vi "DisplayPanel.vi"() -> ()   [LabVIEW 2013]
uses:
  MvLVLib/MvCameraControl.lvlib
  MvLVLib/VIs/CreateGigEHandle.vi
  MvLVLib/VIs/CreateU3VHandle.vi
panel:
  out "GenTLDeviceArray":T1(array[cluster])
  out "Image":T2(plugin-control)
  out "U3VDeviceArray":T3(array[cluster])
  out "GigEDeviceArray":T4(array[cluster])
  in  "pConvertInfo In":T5
  out "PixelFormat":u32
  out "handle out":u64
  out "PayloadSize":u32
  out "pFrameInfoEx out":T6
  out "nHeight":u32
  out "nWidth":u32
  out "Acquisision Flag":bool
  in  "Trigger Mode":bool
  in  "Continuous":bool
  out "打开标志":bool
  in  "stop":bool
  in  "Trigger Once":bool
  in  "Stop":bool
  in  "Start":bool
  in  "Open Device":bool
  in  "Close Device":bool
  in  "error in (no error) 2":errorcluster caption="错误输入（无错误）"
  in  "Refresh Devices":bool
  in  "Device List":u16(ring)
  # "Initialize"
  # "Acquisition"
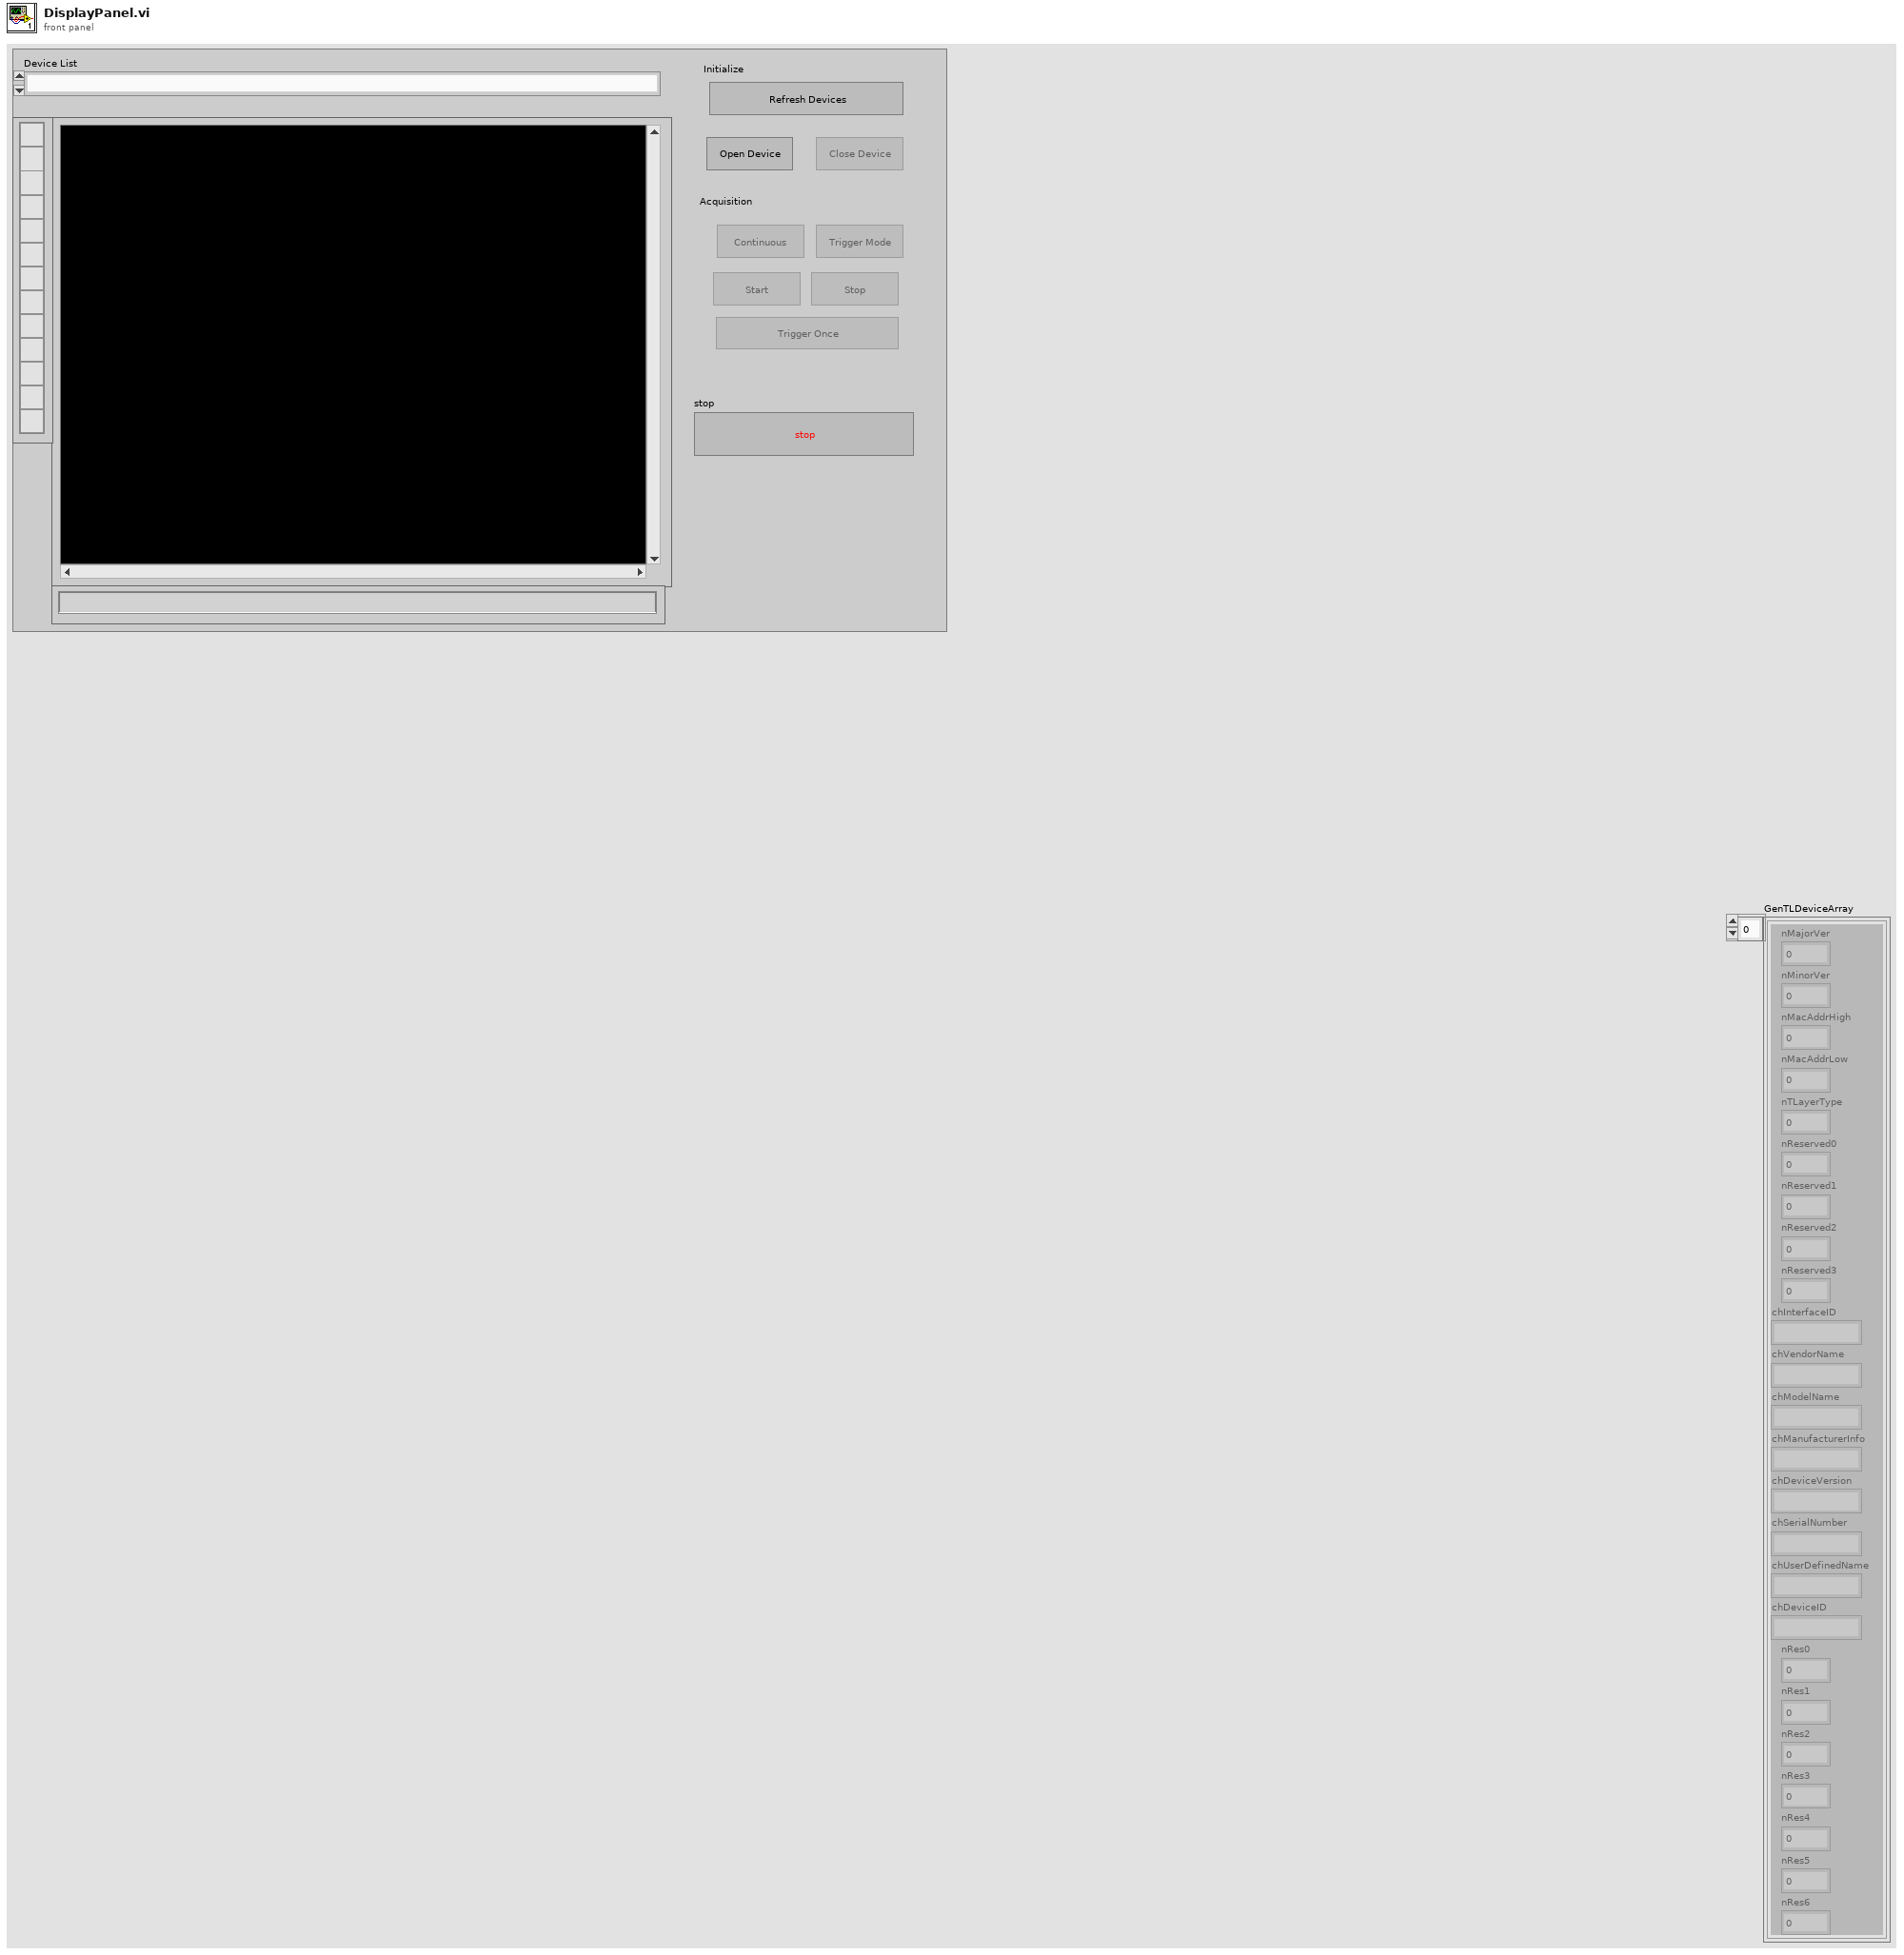
[diagram p1: front panel]
types:
  T1 = cluster{"nMajorVer":u16, "nMinorVer":u16, "nMacAddrHigh":u32, "nMacAddrLow":u32, "nTLayerType":u32, "nReserved0":u32, "nReserved1":u32, "nReserved2":u32, "nReserved3":u32, "chInterfaceID":string, "chVendorName":string, "chModelName":string, "chManufacturerInfo":string, "chDeviceVersion":string, "chSerialNumber":string, "chUserDefinedName":string, "chDeviceID":string, "nRes0":u32, "nRes1":u32, "nRes2":u32, "nRes3":u32, "nRes4":u32, "nRes5":u32, "nRes6":u32}[]
  T2 = typedef "IMAQ Image.ctl" = refnum<image>
  T3 = cluster{"nMajorVer":u16, "nMinorVer":u16, "nMacAddrHigh":u32, "nMacAddrLow":u32, "nTLayerType":u32, "nReserved0":u32, "nReserved1":u32, "nReserved2":u32, "nReserved3":u32, "CrtlInEndPoint":u8, "CrtlOutEndPoint":u8, "StreamEndPoint":u8, "EventEndPoint":u8, "idVendor":u16, "idProduct":u16, "nDeviceNumber":u32, "chDeviceGUID":string, "chVendorName":string, "chModelName":string, "chFamilyName":string, "chDeviceVersion":string, "chManufacturerName":string, "chSerialNumber":string, "chUserDefinedName":string, "nbcdUSB":u32, "nDeviceAddress":u32, "nRes0":u32, "nRes1":u32, "nResAlign":u32}[]
  T4 = cluster{"nMajorVer":u16, "nMinorVer":u16, "nMacAddrHigh":u32, "nMacAddrLow":u32, "nTLayerType":u32, "nReserved0":u32, "nReserved1":u32, "nReserved2":u32, "nReserved3":u32, "nIpCfgOption":u32, "nIpCfgCurrent":u32, "nCurrentIp":u32, "nCurrentSubNetMask":u32, "nDefaultGateWay":u32, "chManualfacturerName":string, "chModelName":string, "chDeviceVersion":string, "chManufacturerSpecificInfo":string, "chSerialNumber":string, "chUserDefinedName":string, "nNetExport":u32, "nRes0":u32, "nRes1":u32, "nRes2":u32, "nRes3":u32}[]
  T5 = cluster{"nWidth":u16, "nHeight":u16, "enSrcPixelType":u32, "nSrcDataLen":u32, "enDstPixelType":u32, "nDstLen":u32, "nDstBufferSize":u32, "nRes0":u32, "nRes1":u32, "nRes2":u32, "nRes3":u32}
  T6 = cluster{"nWidth":u16, "nHeight":u16, "enPixelType":i32, "nFrameNum":u32, "nDevTimeStampHigh":u32, "nDevTimeStampLow":u32, "nReserved0":u32, "nHostTimeStamp":i64, "nFrameLen":u32, "nSecondCount]":u32, "nCycleCount":u32, "nCycleOffset":u32, "fGain":u32, "fExposureTime":u32, "nAverageBrightness":u32, "nRed":u32, "nGreen":u32, "nBlue":u32, "nFrameCounter":u32, "nTriggerIndex":u32, "nInput":u32, "nOutput":u32, "nOffsetX":u32, "nOffsetY":u32, "nReserved[0]":u32, "nReserved[1]":u32, "nReserved[2]":u32, "nReserved[3]":u32, "nReserved[4]":u32, "nReserved[5]":u32, "nReserved[6]":u32, "nReserved[7]":u32, "nReserved[8]":u32, "nReserved[9]":u32, "nReserved[10]":u32, "nReserved[11]":u32, "nReserved[12]":u32, "nReserved[13]":u32, "nReserved[14] 10":u32, "nReserved[15] 11":u32, "nReserved[16] 12":u32, "nReserved[17] 13":u32, "nReserved[18] 14":u32, "nReserved[19] 15":u32, "nReserved[20] 16":u32, "nReserved[21] 17":u32, "nReserved[22] 18":u32, "nReserved[23] 19":u32, "nReserved[24] 20":u32, "nReserved[25] 21":u32, "nReserved[26] 22":u32, "nReserved[27] 23":u32, "nReserved[28] 24":u32, "nReserved[29] 25":u32, "nReserved[30] 26":u32, "nReserved[31] 27":u32, "nReserved[32] 28":u32, "nReserved[33] 29":u32, "nReserved[34] 30":u32, "nReserved[35] 31":u32, "nReserved[36] 32":u32, "nReserved[37] 33":u32, "nReserved[38] 34":u32, "nReserved[39] 35":u32, "nReserved[40] 36":u32}
  T7 = enum8{"Enabled", "Disabled", "Disabled and Grayed Out"}
  T8 = cluster{"nMajorVer":u16, "nMinorVer":u16, "nMacAddrHigh":u32, "nMacAddrLow":u32, "nTLayerType":u32, "nReserved0":u32, "nReserved1":u32, "nReserved2":u32, "nReserved3":u32, "nIpCfgOption":u32, "nIpCfgCurrent":u32, "nCurrentIp":u32, "nCurrentSubNetMask":u32, "nDefaultGateWay":u32, "chManualfacturerName":string, "chModelName":string, "chDeviceVersion":string, "chManufacturerSpecificInfo":string, "chSerialNumber":string, "chUserDefinedName":string, "nNetExport":u32, "nRes0":u32, "nRes1":u32, "nRes2":u32, "nRes3":u32}
  T9 = cluster{"nMajorVer":u16, "nMinorVer":u16, "nMacAddrHigh":u32, "nMacAddrLow":u32, "nTLayerType":u32, "nReserved0":u32, "nReserved1":u32, "nReserved2":u32, "nReserved3":u32, "CrtlInEndPoint":u8, "CrtlOutEndPoint":u8, "StreamEndPoint":u8, "EventEndPoint":u8, "idVendor":u16, "idProduct":u16, "nDeviceNumber":u32, "chDeviceGUID":string, "chVendorName":string, "chModelName":string, "chFamilyName":string, "chDeviceVersion":string, "chManufacturerName":string, "chSerialNumber":string, "chUserDefinedName":string, "nbcdUSB":u32, "nDeviceAddress":u32, "nRes0":u32, "nRes1":u32, "nResAlign":u32}
  T10 = cluster{"nCurValue":u32, "nMax":u32, "nMin":u32, "nInc":u32, "nReserved[0]":u32, "nReserved[1]":u32, "nReserved[2]":u32, "nReserved[3]":u32}
  T11 = cluster{"nCurValue":u32, "nSupportedNum":u32, "nSupportValue":u32[], "nReserved[0]":u32, "nReserved[1]":u32, "nReserved[2]":u32, "nReserved[3]":u32}
  T12 = cluster{"nWidth":u32, "nHeight":u32, "enSrcPixelType":u32, "nSrcDataLen":u32, "enDstPixelType":u32, "nDstLen":u32, "nDstBufferSize":u32, "nRes0":u32, "nRes1":u32, "nRes2":u32, "nRes3":u32}
  T13 = typedef "Image Type" = u32
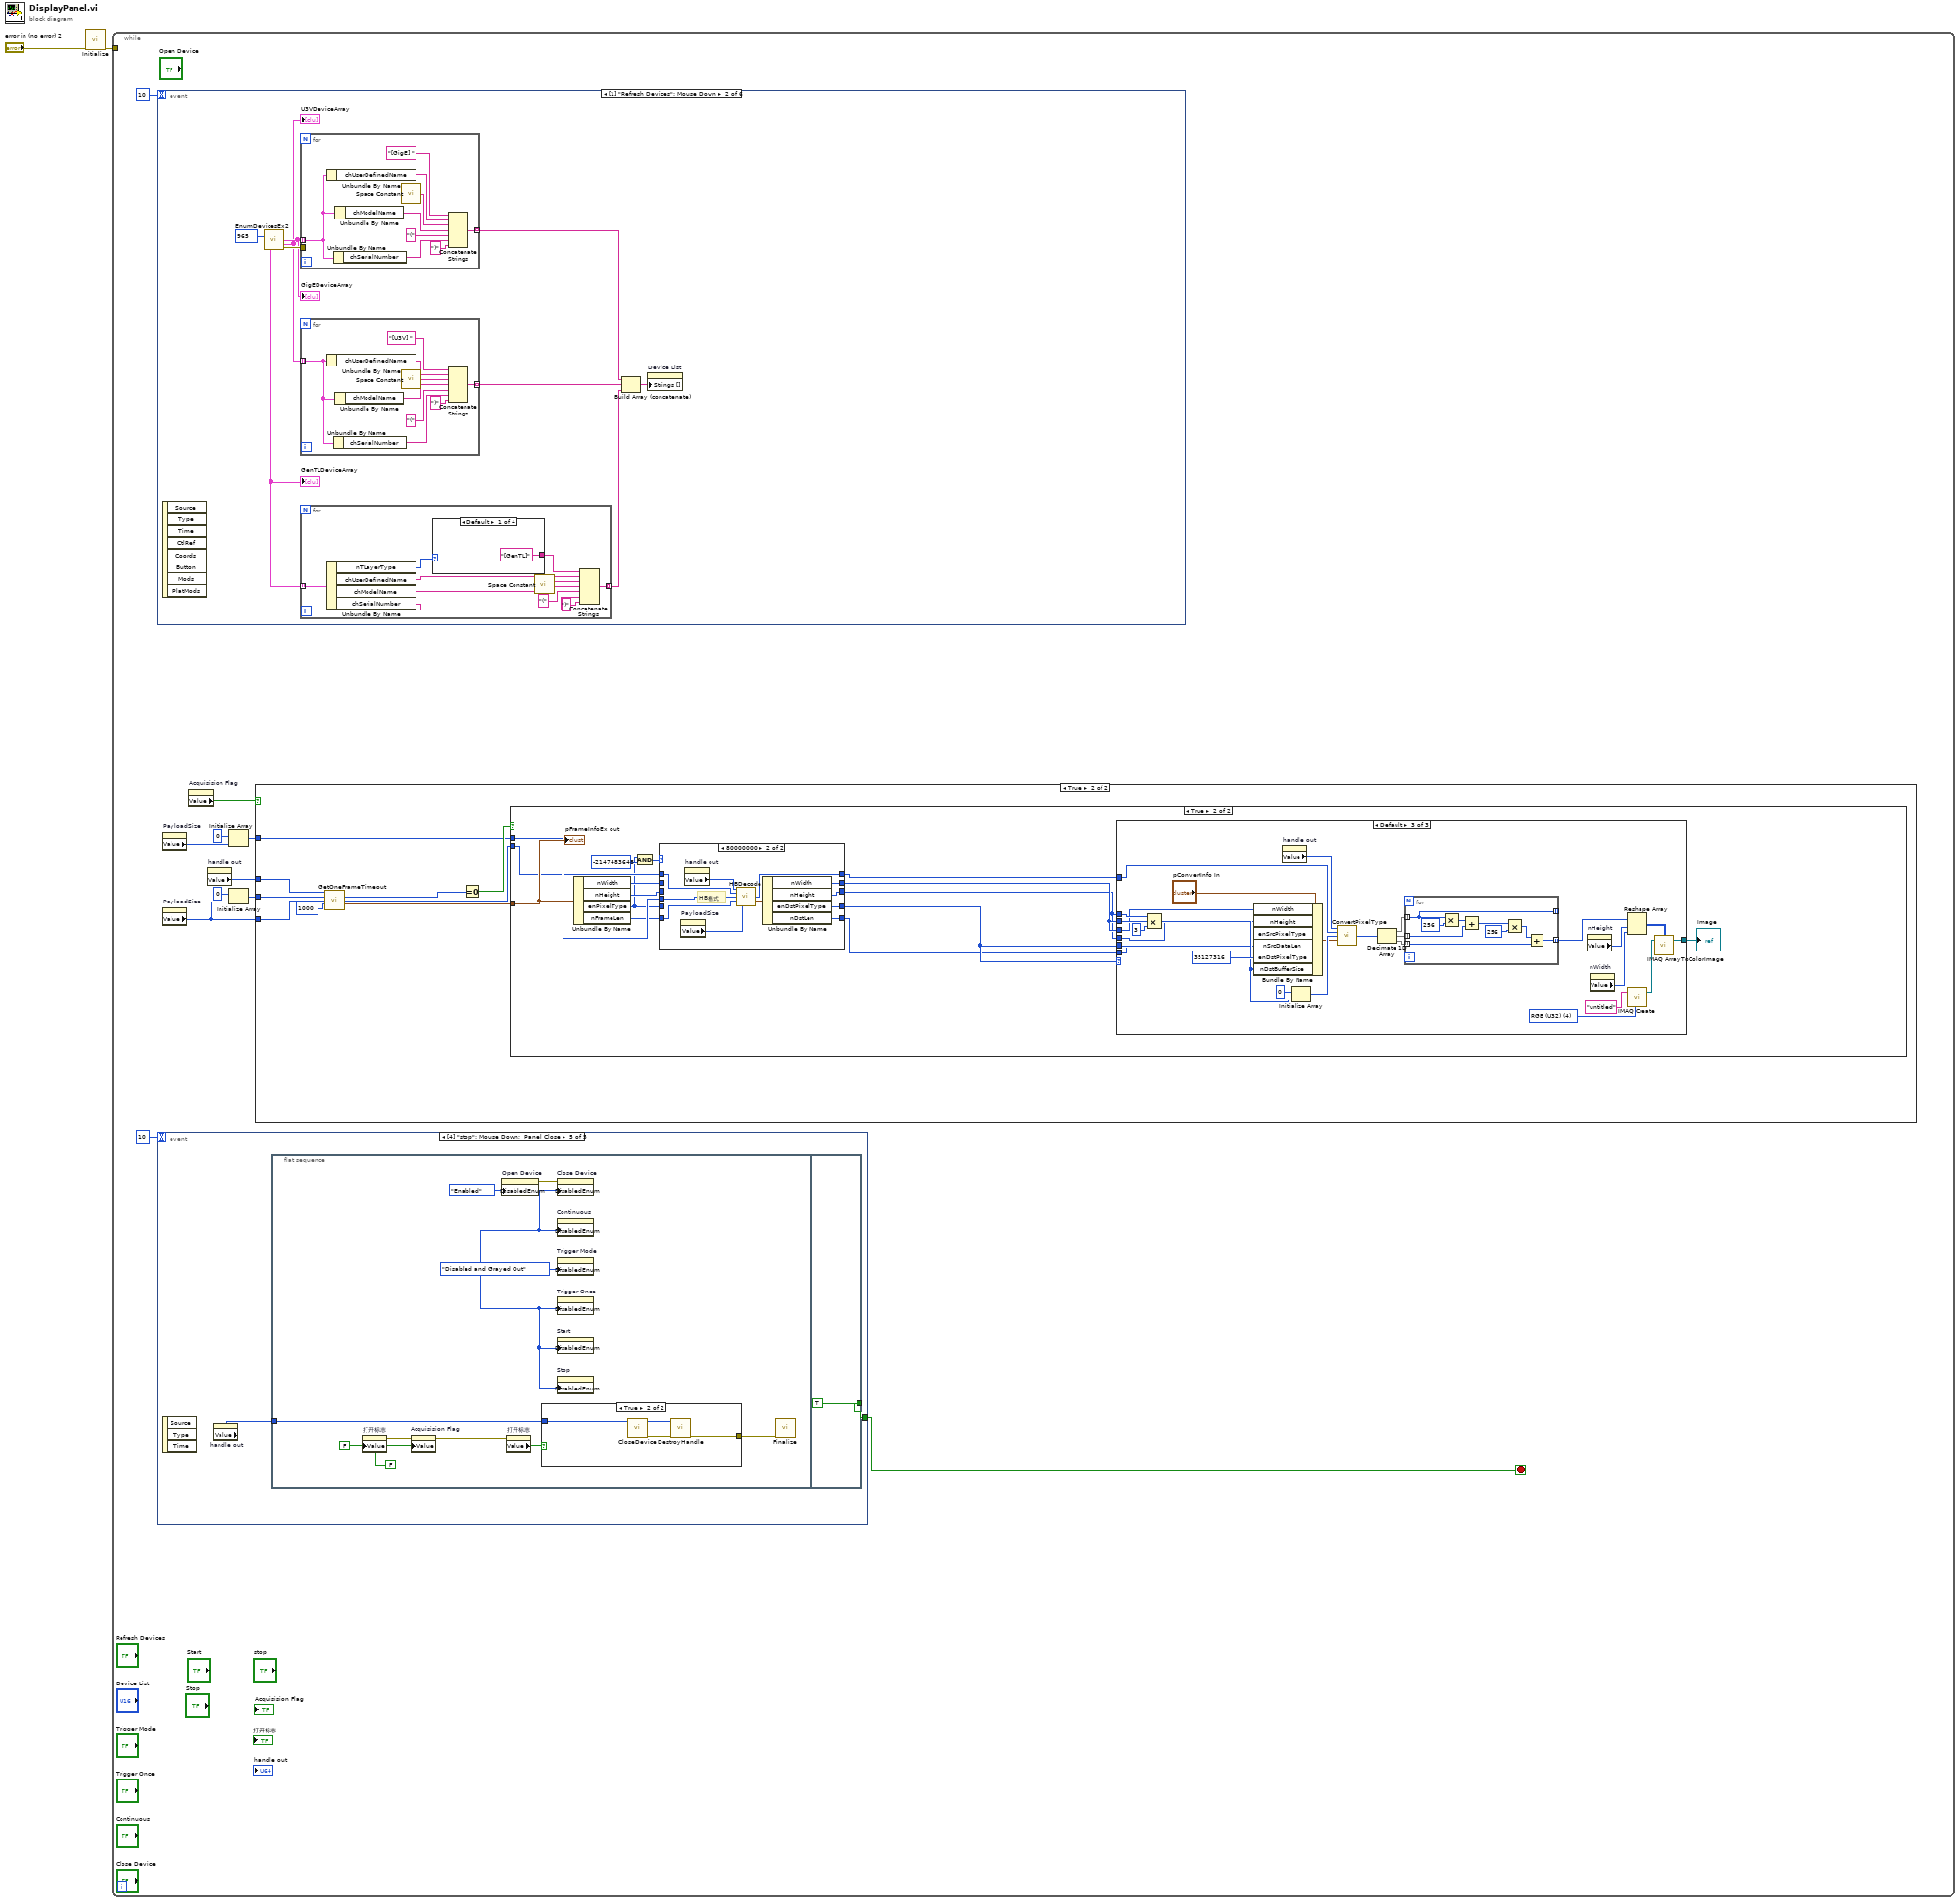
[diagram p0: block diagram]
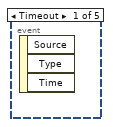
[diagram p2: hidden frame]
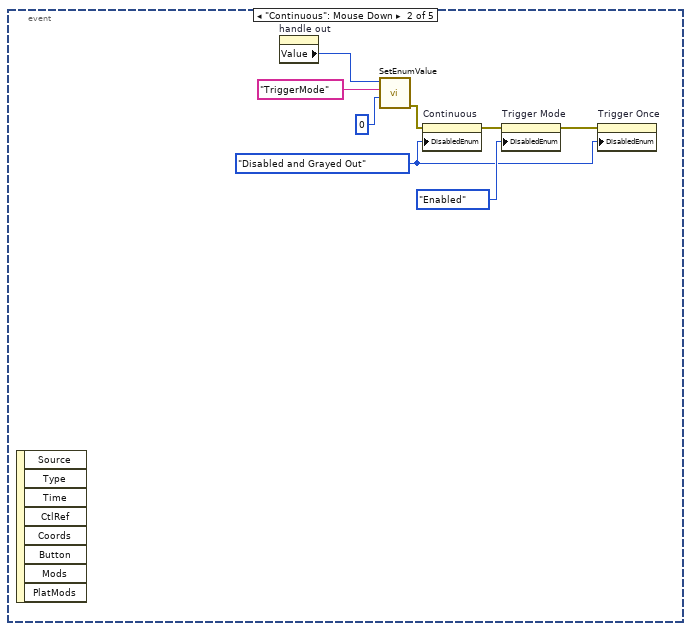
[diagram p3: hidden frame]
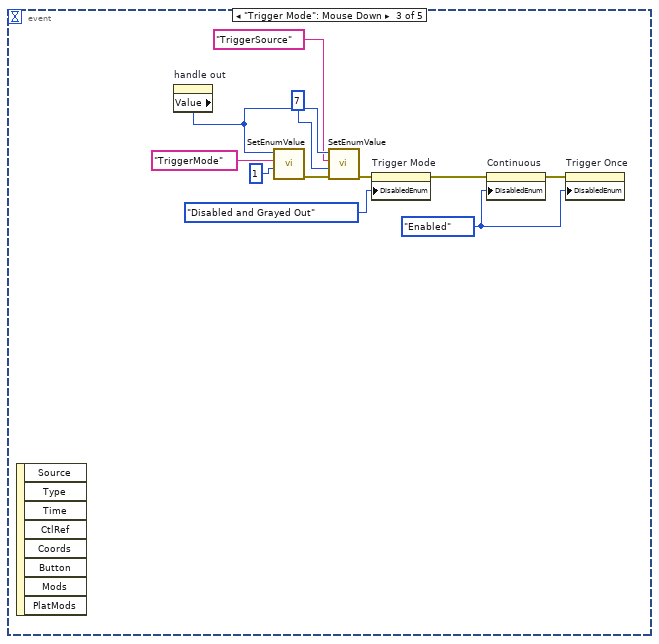
[diagram p4: hidden frame]
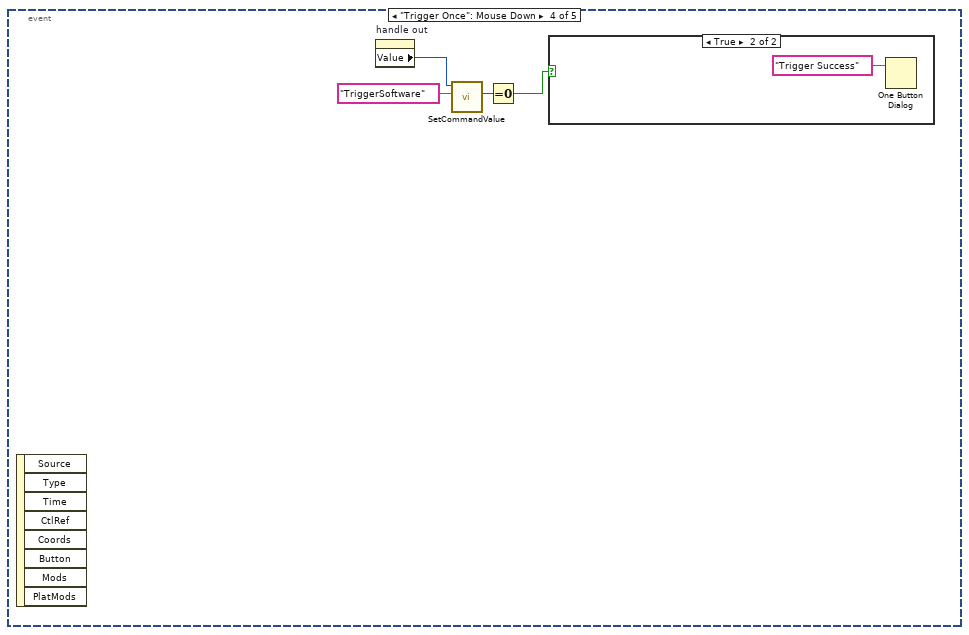
[diagram p5: hidden frame]
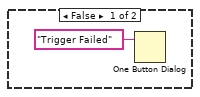
[diagram p6: hidden frame]
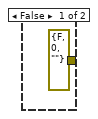
[diagram p7: hidden frame]
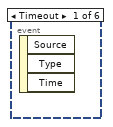
[diagram p8: hidden frame]
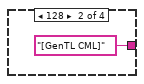
[diagram p9: hidden frame]
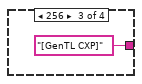
[diagram p10: hidden frame]
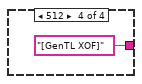
[diagram p11: hidden frame]
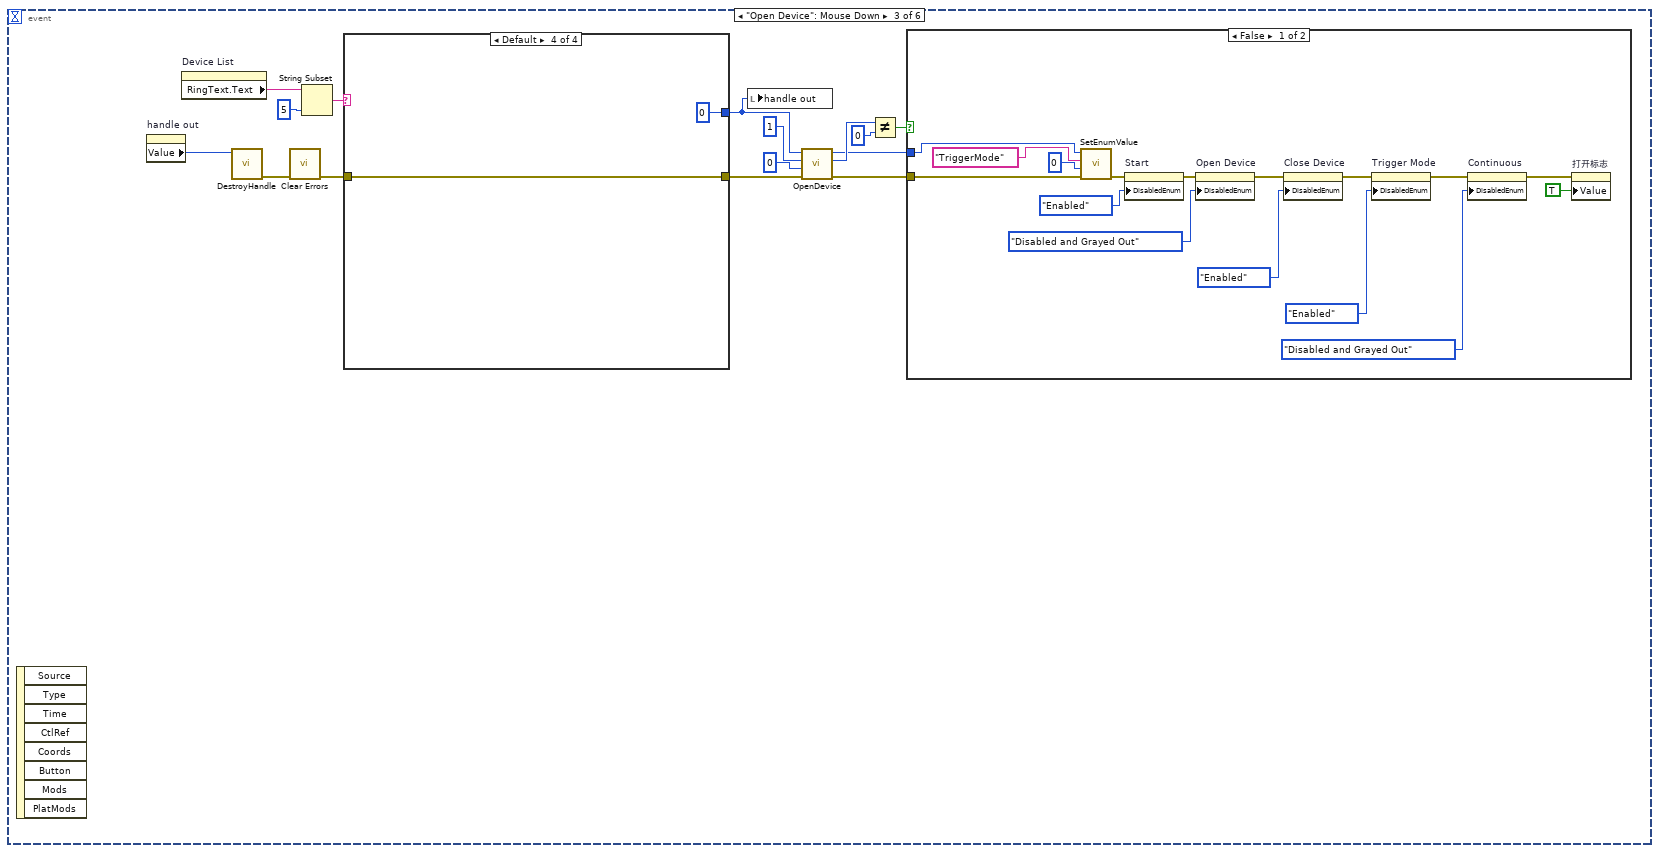
[diagram p12: hidden frame]
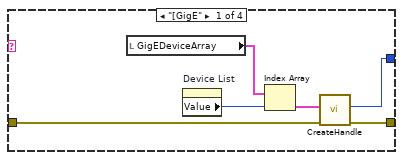
[diagram p13: hidden frame]
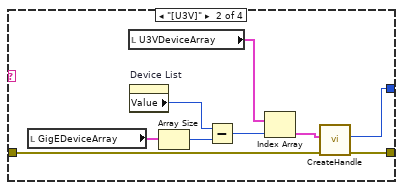
[diagram p14: hidden frame]
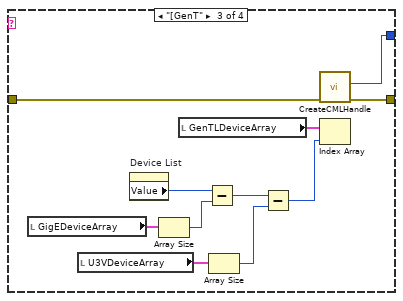
[diagram p15: hidden frame]
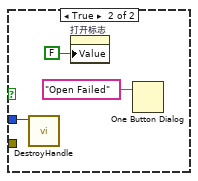
[diagram p16: hidden frame]
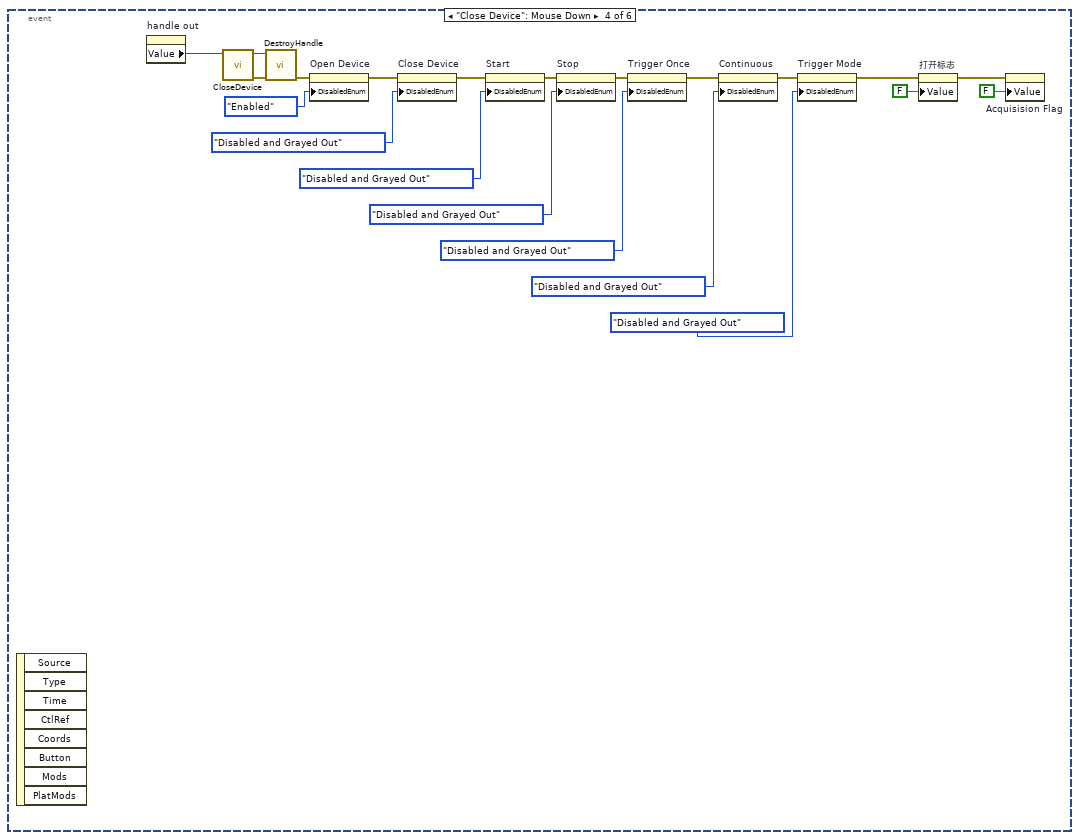
[diagram p17: hidden frame]
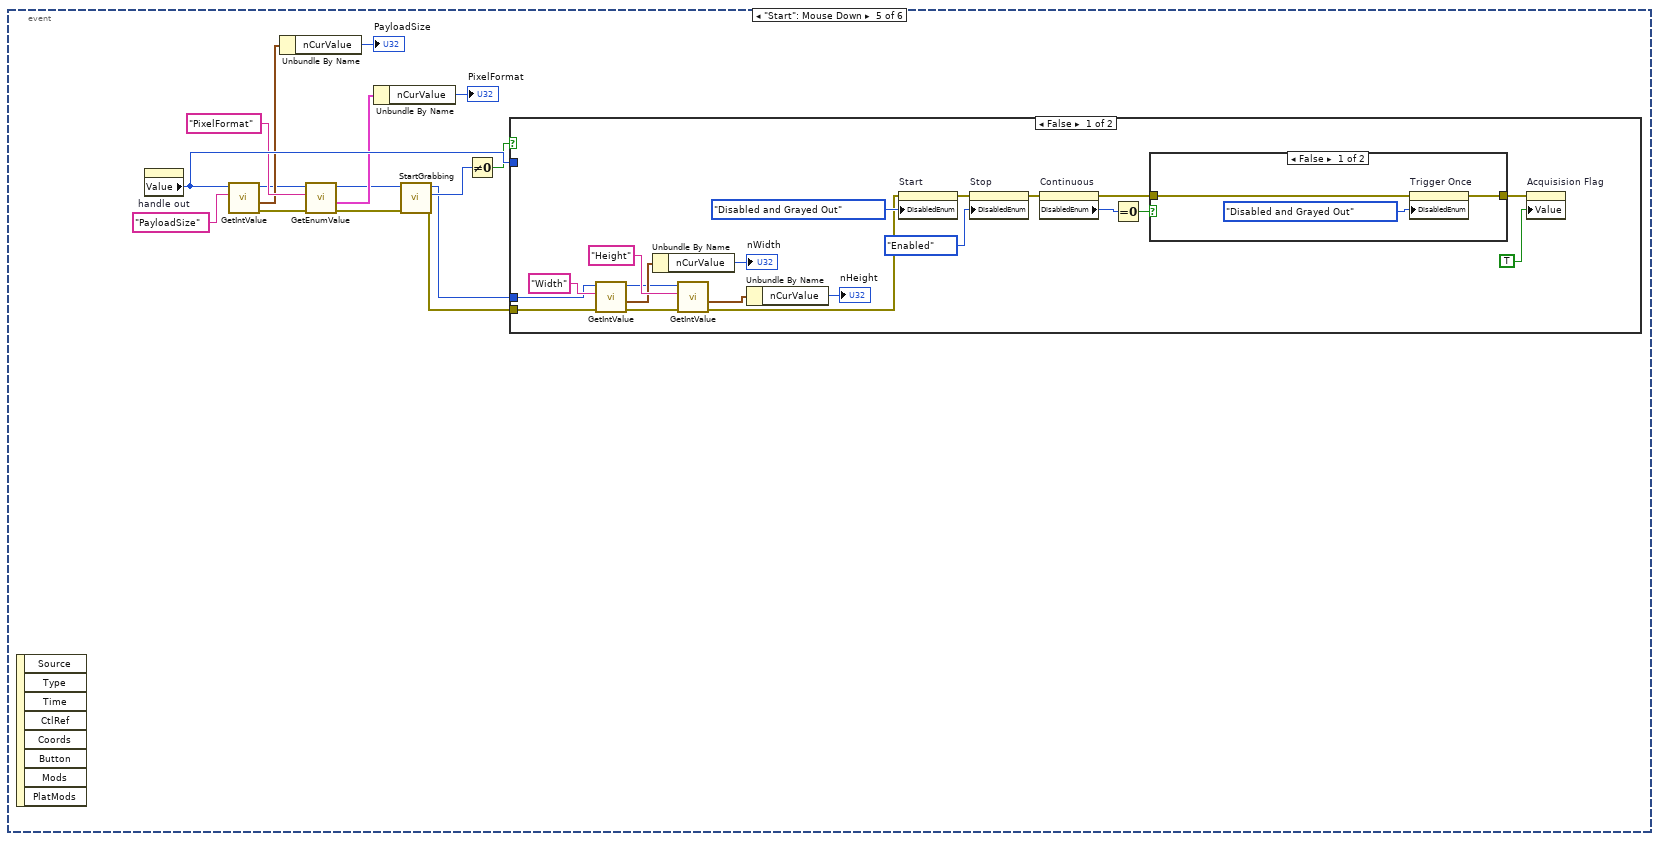
[diagram p18: hidden frame]
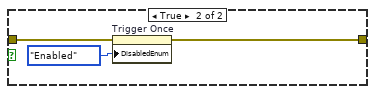
[diagram p19: hidden frame]
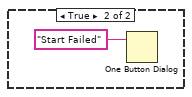
[diagram p20: hidden frame]
diagram:
  n1 = call "Initialize.vi"("error in (no error)"="error in (no error) 2") -> ("error out"=w2:errorcluster)  [unwired: 9 in, 1 out]
  n2 = while {
    tunnel: w2 -> [_]
    stop <- w3 stop-if-true
    n3 = event shown="[1] \"Refresh Devices\": Mouse Down" {
      selector: _ -> [_ _ _ _ _ _]
      dyn-events: _ -> [_ _ _ _ _ _]
      timeout: 10 -> [_ _ _ _ _ _]
      event Timeout {
        n4 = event-data() -> ()  [unwired: 1 in, 3 out]
      }
      event "Refresh Devices": Mouse Down {
        n5 = event-data() -> ()  [unwired: 1 in, 8 out]
        n6 = call "EnumDevicesEx2.vi"("nLayerType"=965) -> ("GigEDeviceArray"=w58:T4, "U3VDeviceArray"=w57:T3, "GenTLDevice"=w64:T1, "error out"=w59:errorcluster)  [unwired: 9 in, 2 out]
        "GenTLDeviceArray" <- w64
        "GigEDeviceArray" <- w58
        "U3VDeviceArray" <- w57
        n7 = for {
          tunnel: w59 -> [_]
          tunnel: w58 -> [w91] mode=indexing
          tunnel: [w90] -> w60 mode=indexing
          n8 = Unbundle By Name(w91) -> ("chUserDefinedName"=w94:string)
          n9 = Unbundle By Name(w91) -> ("chSerialNumber"=w92:string)
          n10 = Unbundle By Name(w91) -> ("chModelName"=w93:string)
          n11 = call <vilib>:"Space Constant.vi"() -> ("String"=w97:string)
          n12 = Concatenate Strings("[GigE] " ("字符串"), w94, w97, w93, "(" ("字符串"), w92, ")" ("字符串")) -> (w90:string)
        }
        n13 = for {
          tunnel: w57 -> [w84] mode=indexing
          tunnel: [w81] -> w61 mode=indexing
          n14 = Unbundle By Name(w84) -> ("chUserDefinedName"=w88:string)
          n15 = Unbundle By Name(w84) -> ("chSerialNumber"=w83:string)
          n16 = Unbundle By Name(w84) -> ("chModelName"=w86:string)
          n17 = call <vilib>:"Space Constant.vi"() -> ("String"=w87:string)
          n18 = Concatenate Strings("[U3V] " ("字符串"), w88, w87, w86, "(" ("字符串"), w83, ")" ("字符串")) -> (w81:string)
        }
        n19 = for {
          tunnel: w64 -> [w72] mode=indexing
          tunnel: [w70] -> w65 mode=indexing
          n20 = Unbundle By Name(w72) -> ("nTLayerType"=w67:u32, "chUserDefinedName"=w75:string, "chModelName"=w69:string, "chSerialNumber"=w68:string)
          n21 = case shown="Default" w67 {
            tunnel: ["[GenTL]" ("字符串") "[GenTL CML]" ("字符串") "[GenTL CXP]" ("字符串") "[GenTL XOF]" ("字符串")] -> w66
            frame Default {
            }
            frame 128 {
            }
            frame 256 {
            }
            frame 512 {
            }
          }
          n22 = call <vilib>:"Space Constant.vi"() -> ("String"=w74:string)
          n23 = Concatenate Strings(w66, w75, w74, w69, "(" ("字符串"), w68, ")" ("字符串")) -> (w70:string)
        }
        n24 = Build Array (concatenate)(w60, w61, w65) -> (w62:string[])
        n25 = property on="Device List" class="Ring (strict)"("Strings []"=w62) -> ()  [unwired: 2 in, 2 out]
      }
      event "Open Device": Mouse Down {
        n26 = event-data() -> ()  [unwired: 1 in, 8 out]
        n27 = property on="handle out" class="DigNum (strict)"() -> ("Value"=w102:u64)  [unwired: 2 in, 2 out]
        n28 = property on="Device List" class="Ring (strict)"() -> ("RingText.Text"=w106:string)  [unwired: 2 in, 2 out]
        n29 = call "DestroyHandle.vi"("handle"=w102) -> ("error out"=w101:errorcluster)  [unwired: 9 in, 1 out]
        n30 = call <vilib>:"Clear Errors.vi"("error in (no error)"=w101) -> ("error out"=w100:errorcluster)  [unwired: 5 in, 1 out]
        n31 = String Subset(string=w106, length (rest)=5 ("长度（剩余）")) -> (substring=w99:string)  [unwired: 1 in]
        n32 = case shown="Default" w99 {
          tunnel: [w116 w123 w135 w140] -> w110
          tunnel: [w115 w122 w134 u64 0 ("handle")] -> w98
          tunnel: w100 -> [w117 w124 w136 w140]
          frame "[GigE" {
            n33 = local read "GigEDeviceArray"() -> (w114:T4)
            n34 = property on="Device List" class="Ring (strict)"() -> ("Value"=w118:u16)  [unwired: 2 in, 2 out]
            n35 = Index Array(array=w114, index=w118) -> (element=w113:T8)
            n36 = call-poly "CreateHandle.vi"("error in (no error)"=w117, "GigEDevice"=w113) -> ("error out"=w116:errorcluster, "handle"=w115:u64)  [unwired: 6 in, 1 out]
          }
          frame "[U3V]" {
            n37 = local read "GigEDeviceArray"() -> (w120:T4)
            n38 = local read "U3VDeviceArray"() -> (w121:T3)
            n39 = property on="Device List" class="Ring (strict)"() -> ("Value"=w127:u16)  [unwired: 2 in, 2 out]
            n40 = Array Size(array=w120) -> (size(s)=w126:i32)
            n41 = Subtract(x=w127, y=w126) -> (x-y=w125:i32)
            n42 = Index Array(array=w121, index=w125) -> (element=w119:T9)
            n43 = call-poly "CreateHandle.vi"("error in (no error)"=w124, "U3VDevice"=w119) -> ("error out"=w123:errorcluster, "handle"=w122:u64)  [unwired: 6 in, 1 out]
          }
          frame "[GenT" {
            n44 = local read "GigEDeviceArray"() -> (w133:T4)
            n45 = local read "U3VDeviceArray"() -> (w132:T3)
            n46 = property on="Device List" class="Ring (strict)"() -> ("Value"=w138:u16)  [unwired: 2 in, 2 out]
            n47 = Array Size(array=w133) -> (size(s)=w137:i32)
            n48 = local read "GenTLDeviceArray"() -> (w128:T1)
            n49 = Subtract(x=w138, y=w137) -> (x-y=w131:i32)
            n50 = Array Size(array=w132) -> (size(s)=w130:i32)
            n51 = Subtract(x=w131, y=w130) -> (x-y=w129:i32)
            n52 = call "CreateCMLHandle.vi"("error in (no error)"=w136) -> ("error out"=w135:errorcluster, "handle"=w134:u64)  [unwired: 7 in, 1 out]
            n53 = Index Array(array=w128, index=w129) -> ()  [unwired: 1 out]
          }
          frame Default {
          }
        }
        n54 = local write "handle out"(w98) -> ()
        n55 = call "OpenDevice.vi"("error in (no error)"=w110, "nSwitchoverKey"=u16 0, "nAccessMode"=u32 1, "handle"=w98) -> ("error out"=w107:errorcluster, "return"=w104:i32, "handle out"=w103:u64)  [unwired: 5 in]
        n56 = Not Equal?(x=w104, y=0) -> (x != y?=w111:bool)
        n57 = case shown="False" w111 {
          tunnel: w103 -> [w141 w157]
          tunnel: w107 -> [w142 _]
          frame False {
            n58 = call "SetEnumValue.vi"("error in (no error)"=w142, "nValue"=u32 0, "strKey"="TriggerMode", "handle"=w141) -> ("error out"=w153:errorcluster)  [unwired: 5 in, 2 out]
            n59 = property on="Start" class="Bool"(error in=w153, "DisabledEnum"=T7."Enabled" ("禁用")) -> (error out=w151:errorcluster)  [unwired: 1 in, 1 out]
            n60 = property on="Open Device" class="Bool"(error in=w151, "DisabledEnum"=T7."Disabled and Grayed Out" ("禁用")) -> (error out=w150:errorcluster)  [unwired: 1 in, 1 out]
            n61 = property on="Close Device" class="Bool"(error in=w150, "DisabledEnum"=T7."Enabled" ("禁用")) -> (error out=w147:errorcluster)  [unwired: 1 in, 1 out]
            n62 = property on="Trigger Mode" class="Bool"(error in=w147, "DisabledEnum"=T7."Enabled" ("禁用")) -> (error out=w145:errorcluster)  [unwired: 1 in, 1 out]
            n63 = property on="Continuous" class="Bool"(error in=w145, "DisabledEnum"=T7."Disabled and Grayed Out" ("禁用")) -> (error out=w143:errorcluster)  [unwired: 1 in, 1 out]
            n64 = property on="打开标志" class="Bool (strict)"(error in=w143, "Value"=TRUE ("布尔")) -> ()  [unwired: 1 in, 2 out]
          }
          frame True {
            n65 = call "DestroyHandle.vi"("handle"=w157) -> ()  [unwired: 9 in, 2 out]
            n66 = property on="打开标志" class="Bool (strict)"("Value"=FALSE) -> ()  [unwired: 2 in, 2 out]
            n67 = One Button Dialog(message="Open Failed") -> ()  [unwired: 1 in, 1 out]
          }
        }
      }
      event "Close Device": Mouse Down {
        n68 = event-data() -> ()  [unwired: 1 in, 8 out]
        n69 = property on="handle out" class="DigNum (strict)"() -> ("Value"=w180:u64)  [unwired: 2 in, 2 out]
        n70 = call "CloseDevice.vi"("handle"=w180) -> ("error out"=w162:errorcluster, "handle out"=w160:u64)  [unwired: 8 in, 1 out]
        n71 = call "DestroyHandle.vi"("error in (no error)"=w162, "handle"=w160) -> ("error out"=w161:errorcluster)  [unwired: 8 in, 1 out]
        n72 = property on="Open Device" class="Bool"(error in=w161, "DisabledEnum"=T7."Enabled" ("禁用")) -> (error out=w175:errorcluster)  [unwired: 1 in, 1 out]
        n73 = property on="Close Device" class="Bool"(error in=w175, "DisabledEnum"=T7."Disabled and Grayed Out" ("禁用")) -> (error out=w174:errorcluster)  [unwired: 1 in, 1 out]
        n74 = property on="Start" class="Bool"(error in=w174, "DisabledEnum"=T7."Disabled and Grayed Out" ("禁用")) -> (error out=w173:errorcluster)  [unwired: 1 in, 1 out]
        n75 = property on="Stop" class="Bool"(error in=w173, "DisabledEnum"=T7."Disabled and Grayed Out" ("禁用")) -> (error out=w172:errorcluster)  [unwired: 1 in, 1 out]
        n76 = property on="Trigger Once" class="Bool"(error in=w172, "DisabledEnum"=T7."Disabled and Grayed Out" ("禁用")) -> (error out=w169:errorcluster)  [unwired: 1 in, 1 out]
        n77 = property on="Continuous" class="Bool"(error in=w169, "DisabledEnum"=T7."Disabled and Grayed Out" ("禁用")) -> (error out=w167:errorcluster)  [unwired: 1 in, 1 out]
        n78 = property on="Trigger Mode" class="Bool"(error in=w167, "DisabledEnum"=T7."Disabled and Grayed Out" ("禁用")) -> (error out=w166:errorcluster)  [unwired: 1 in, 1 out]
        n79 = property on="打开标志" class="Bool (strict)"(error in=w166, "Value"=FALSE ("打开标志")) -> (error out=w164:errorcluster)  [unwired: 1 in, 1 out]
        n80 = property on="Acquisision Flag" class="Bool (strict)"(error in=w164, "Value"=FALSE ("采集标志")) -> ()  [unwired: 1 in, 2 out]
      }
      event "Start": Mouse Down {
        n81 = event-data() -> ()  [unwired: 1 in, 8 out]
        n82 = property on="handle out" class="DigNum (strict)"() -> ("Value"=w195:u64)  [unwired: 2 in, 2 out]
        n83 = call "GetIntValue.vi"("strKey"="PayloadSize", "handle"=w195) -> ("error out"=w190:errorcluster, "pIntValue out"=w186:T10, "handle out"=w183:u64)  [unwired: 6 in, 1 out]
        n84 = Unbundle By Name(w186) -> ("nCurValue"=→"PayloadSize":u32)
        n85 = call "GetEnumValue.vi"("error in (no error)"=w190, "strKey"="PixelFormat", "handle"=w183) -> ("error out"=w189:errorcluster, "pEnumValue out"=w191:T11, "handle out"=w182:u64)  [unwired: 5 in, 1 out]
        n86 = Unbundle By Name(w191) -> ("nCurValue"=→"PixelFormat":u32)
        n87 = call "StartGrabbing.vi"("error in (no error)"=w189, "handle"=w182) -> ("error out"=w188:errorcluster, "function return"=w194:i32, "handle out"=w181:u64)  [unwired: 7 in]
        n88 = Not Equal To 0?(x=w194) -> (x != 0?=w193:bool)
        n89 = case shown="False" w193 {
          tunnel: w195 -> [_ _]
          tunnel: w188 -> [w198 _]
          tunnel: w181 -> [w197 _]
          frame False {
            n90 = call "GetIntValue.vi"("error in (no error)"=w198, "strKey"="Width", "handle"=w197) -> ("error out"=w205:errorcluster, "pIntValue out"=w199:T10, "handle out"=w196:u64)  [unwired: 5 in, 1 out]
            n91 = Unbundle By Name(w199) -> ("nCurValue"=→"nWidth":u32)
            n92 = call "GetIntValue.vi"("error in (no error)"=w205, "strKey"="Height", "handle"=w196) -> ("error out"=w204:errorcluster, "pIntValue out"=w202:T10)  [unwired: 5 in, 2 out]
            n93 = Unbundle By Name(w202) -> ("nCurValue"=→"nHeight":u32)
            n94 = property on="Start" class="Bool"(error in=w204, "DisabledEnum"=T7."Disabled and Grayed Out" ("禁用")) -> (error out=w214:errorcluster)  [unwired: 1 in, 1 out]
            n95 = property on="Stop" class="Bool"(error in=w214, "DisabledEnum"=T7."Enabled" ("禁用")) -> (error out=w200:errorcluster)  [unwired: 1 in, 1 out]
            n96 = property on="Continuous" class="Bool"(error in=w200) -> (error out=w210:errorcluster, "DisabledEnum"=w211:T7)  [unwired: 1 in, 1 out]
            n97 = Equal To 0?(x=w211) -> (x = 0?=w212:bool)
            n98 = case shown="False" w212 {
              tunnel: w210 -> [w217 w220]
              tunnel: [w216 w219] -> w209
              frame False {
                n99 = property on="Trigger Once" class="Bool"(error in=w217, "DisabledEnum"=T7."Disabled and Grayed Out" ("禁用")) -> (error out=w216:errorcluster)  [unwired: 1 in, 1 out]
              }
              frame True {
                n100 = property on="Trigger Once" class="Bool"(error in=w220, "DisabledEnum"=T7."Enabled" ("禁用")) -> (error out=w219:errorcluster)  [unwired: 1 in, 1 out]
              }
            }
            n101 = property on="Acquisision Flag" class="Bool (strict)"(error in=w209, "Value"=TRUE ("采集标志")) -> ()  [unwired: 1 in, 2 out]
          }
          frame True {
            n102 = One Button Dialog(message="Start Failed") -> ()  [unwired: 1 in, 1 out]
          }
        }
      }
      event "Stop": Mouse Down {
        n103 = event-data() -> ()  [unwired: 1 in, 8 out]
        n104 = property on="handle out" class="DigNum (strict)"() -> ("Value"=w231:u64)  [unwired: 2 in, 2 out]
        n105 = call "StopGrabbing.vi"("handle"=w231) -> ("error out"=w230:errorcluster)  [unwired: 8 in, 2 out]
        n106 = property on="Acquisision Flag" class="Bool (strict)"(error in=w230, "Value"=FALSE ("采集标志")) -> (error out=w225:errorcluster)  [unwired: 1 in, 1 out]
        n107 = property on="Start" class="Bool"(error in=w225, "DisabledEnum"=T7."Enabled" ("禁用")) -> (error out=w224:errorcluster)  [unwired: 1 in, 1 out]
        n108 = property on="Stop" class="Bool"(error in=w224, "DisabledEnum"=T7."Disabled and Grayed Out" ("禁用")) -> (error out=w223:errorcluster)  [unwired: 1 in, 1 out]
        n109 = property on="Trigger Once" class="Bool"(error in=w223, "DisabledEnum"=T7."Disabled and Grayed Out" ("禁用")) -> ()  [unwired: 1 in, 2 out]
      }
    }
    n110 = event shown="[4] \"stop\": Mouse Down;  Panel Close" {
      selector: _ -> [_ _ _ _ _]
      dyn-events: _ -> [_ _ _ _ _]
      timeout: 10 -> [_ _ _ _ _]
      tunnel: [_ _ _ _ w39] -> w3
      event Timeout {
        n111 = event-data() -> ()  [unwired: 1 in, 3 out]
      }
      event "Continuous": Mouse Down {
        w14 = T7."Disabled and Grayed Out" ("禁用")
        n112 = event-data() -> ()  [unwired: 1 in, 8 out]
        n113 = property on="handle out" class="DigNum (strict)"() -> ("Value"=w21:u64)  [unwired: 2 in, 2 out]
        n114 = call "SetEnumValue.vi"("nValue"=u32 0, "strKey"="TriggerMode", "handle"=w21) -> ("error out"=w15:errorcluster)  [unwired: 6 in, 2 out]
        n115 = property on="Continuous" class="Bool"(error in=w15, "DisabledEnum"=w14) -> (error out=w18:errorcluster)  [unwired: 1 in, 1 out]
        n116 = property on="Trigger Mode" class="Bool"(error in=w18, "DisabledEnum"=T7."Enabled" ("禁用")) -> (error out=w16:errorcluster)  [unwired: 1 in, 1 out]
        n117 = property on="Trigger Once" class="Bool"(error in=w16, "DisabledEnum"=w14) -> ()  [unwired: 1 in, 2 out]
      }
      event "Trigger Mode": Mouse Down {
        w22 = T7."Enabled" ("禁用")
        n118 = event-data() -> ()  [unwired: 1 in, 8 out]
        n119 = property on="handle out" class="DigNum (strict)"() -> ("Value"=w32:u64)  [unwired: 2 in, 2 out]
        n120 = call "SetEnumValue.vi"("nValue"=u32 1, "strKey"="TriggerMode", "handle"=w32) -> ("error out"=w26:errorcluster)  [unwired: 6 in, 2 out]
        n121 = call "SetEnumValue.vi"("error in (no error)"=w26, "nValue"=u32 7, "strKey"="TriggerSource", "handle"=w32) -> ("error out"=w25:errorcluster)  [unwired: 5 in, 2 out]
        n122 = property on="Trigger Mode" class="Bool"(error in=w25, "DisabledEnum"=T7."Disabled and Grayed Out" ("禁用")) -> (error out=w24:errorcluster)  [unwired: 1 in, 1 out]
        n123 = property on="Continuous" class="Bool"(error in=w24, "DisabledEnum"=w22) -> (error out=w23:errorcluster)  [unwired: 1 in, 1 out]
        n124 = property on="Trigger Once" class="Bool"(error in=w23, "DisabledEnum"=w22) -> ()  [unwired: 1 in, 2 out]
      }
      event "Trigger Once": Mouse Down {
        n125 = event-data() -> ()  [unwired: 1 in, 8 out]
        n126 = property on="handle out" class="DigNum (strict)"() -> ("Value"=w36:u64)  [unwired: 2 in, 2 out]
        n127 = call "SetCommandValue.vi"("strValue"="TriggerSoftware", "handle"=w36) -> ("function return"=w34:i32)  [unwired: 7 in, 2 out]
        n128 = Equal To 0?(x=w34) -> (x = 0?=w33:bool)
        n129 = case shown="True" w33 {
          frame False {
            n130 = One Button Dialog(message="Trigger Failed") -> ()  [unwired: 1 in, 1 out]
          }
          frame True {
            n131 = One Button Dialog(message="Trigger Success") -> ()  [unwired: 1 in, 1 out]
          }
        }
      }
      event "stop": Mouse Down; Panel Close {
        n132 = event-data() -> ()  [unwired: 1 in, 3 out]
        n133 = property on="handle out" class="DigNum (strict)"() -> ("Value"=w40:u64)  [unwired: 2 in, 2 out]
        n134 = flat-sequence {
          tunnel: w40 -> [w44]
          tunnel: [TRUE] -> w39
          frame #0 {
            w42 = T7."Disabled and Grayed Out" ("禁用")
            n135 = property on="打开标志" class="Bool (strict)"("Value"=FALSE ("打开标志")) -> (error out=w45:errorcluster)  [unwired: 2 in, 1 out]
            n136 = property on="Acquisision Flag" class="Bool (strict)"(error in=w45, "Value"=FALSE ("采集标志")) -> (error out=w41:errorcluster)  [unwired: 1 in, 1 out]
            n137 = property on="Open Device" class="Bool"("DisabledEnum"=T7."Enabled" ("禁用")) -> (error out=w49:errorcluster)  [unwired: 2 in, 1 out]
            n138 = property on="打开标志" class="Bool (strict)"(error in=w41) -> ("Value"=w48:bool)  [unwired: 1 in, 2 out]
            n139 = case shown="True" w48 {
              tunnel: w44 -> [_ w53]
              tunnel: [errorcluster {"status"=FALSE, "code"=0, "source"=""} ("error out") w52] -> w43
              frame False {
              }
              frame True {
                n140 = call "CloseDevice.vi"("handle"=w53) -> ("error out"=w55:errorcluster, "handle out"=w54:u64)  [unwired: 8 in, 1 out]
                n141 = call "DestroyHandle.vi"("error in (no error)"=w55, "handle"=w54) -> ("error out"=w52:errorcluster)  [unwired: 8 in, 1 out]
              }
            }
            n142 = property on="Close Device" class="Bool"(error in=w49, "DisabledEnum"=w42) -> ()  [unwired: 1 in, 2 out]
            n143 = property on="Continuous" class="Bool"("DisabledEnum"=w42) -> ()  [unwired: 2 in, 2 out]
            n144 = property on="Trigger Mode" class="Bool"("DisabledEnum"=w42) -> ()  [unwired: 2 in, 2 out]
            n145 = property on="Trigger Once" class="Bool"("DisabledEnum"=w42) -> ()  [unwired: 2 in, 2 out]
            n146 = property on="Start" class="Bool"("DisabledEnum"=w42) -> ()  [unwired: 2 in, 2 out]
            n147 = property on="Stop" class="Bool"("DisabledEnum"=w42) -> ()  [unwired: 2 in, 2 out]
            n148 = call "Finalize.vi"("error in (no error)"=w43) -> ()  [unwired: 9 in, 2 out]
          }
          frame #1 {
          }
        }
      }
    }
    n149 = property on="PayloadSize" class="DigNum (strict)"() -> ("Value"=w8:u32)  [unwired: 2 in, 2 out]
    n150 = property on="PayloadSize" class="DigNum (strict)"() -> ("Value"=w9:u32)  [unwired: 2 in, 2 out]
    n151 = property on="Acquisision Flag" class="Bool (strict)"() -> ("Value"=w13:bool)  [unwired: 2 in, 2 out]
    n152 = property on="handle out" class="DigNum (strict)"() -> ("Value"=w12:u64)  [unwired: 2 in, 2 out]
    n153 = Initialize Array(u8 0 ("元素"), w8) -> (w6:u8[])
    n154 = Initialize Array(u8 0 ("元素"), w9) -> (w10:u8[])
    n155 = case shown="True" w13 {
      tunnel: w12 -> [_ w238]
      tunnel: w10 -> [_ w237]
      tunnel: w9 -> [_ w236]
      tunnel: w6 -> [_ w232]
      frame False {
      }
      frame True {
        n156 = call "GetOneFrameTimeout.vi"("handle"=w238, "pData"=w237, "nDataSize"=w236, "nMsec"=1000) -> ("function return"=w235:i32, "pData Out"=w234:u8[], "pFrameInfoEx out"=w233:T6)  [unwired: 7 in, 2 out]
        n157 = Equal To 0?(x=w235) -> (x = 0?=w240:bool)
        n158 = case shown="True" w240 {
          tunnel: w234 -> [_ w250]
          tunnel: w233 -> [_ w254]
          tunnel: w232 -> [_ w251]
          frame False {
          }
          frame True {
            n159 = Unbundle By Name(w254) -> ("nWidth"=w243:u16, "nHeight"=w242:u16, "enPixelType"=w241:i32, "nFrameLen"=w249:u32)
            n160 = Compound Arithmetic op=AND(w241, -2147483648 ("value")) -> (w252:i32)
            n161 = case shown="80000000" w252 {
              tunnel: w251 -> [_ w270]
              tunnel: w250 -> [w260 w269]
              tunnel: w249 -> [w257 w268]
              tunnel: [w260 w265] -> w248
              tunnel: [w259 w264] -> w247
              tunnel: [w258 w263] -> w246
              tunnel: [w256 w262] -> w245
              tunnel: [w257 w261] -> w244
              tunnel: w243 -> [w259 _]
              tunnel: w242 -> [w258 _]
              tunnel: w241 -> [w256 _]
              frame Default {
              }
              frame -2147483648 {
                # "HB格式"
                n162 = property on="PayloadSize" class="DigNum (strict)"() -> ("Value"=w267:u32)  [unwired: 2 in, 2 out]
                n163 = property on="handle out" class="DigNum (strict)"() -> ("Value"=w271:u64)  [unwired: 2 in, 2 out]
                n164 = call "HBDecode.vi"("handle"=w271, "pSrcData"=w269, "pDstBuf In"=w270, "SrcDataLen"=w268, "DstBufferSize"=w267) -> ("pDstBuf Out"=w265:u8[], "pHBDecode Out"=w266:T12)  [unwired: 6 in, 3 out]
                n165 = Unbundle By Name(w266) -> ("nWidth"=w264:u32, "nHeight"=w263:u32, "enDstPixelType"=w262:u32, "nDstLen"=w261:u32)
              }
            }
            n166 = case shown="Default" w245 {
              tunnel: w248 -> [w272 w283 w301]
              tunnel: w246 -> [_ _ w322]
              tunnel: w247 -> [_ _ w321]
              tunnel: [w273 w282 w306] -> w255
              tunnel: w247 -> [_ _ w305]
              tunnel: w246 -> [_ _ w304]
              tunnel: w245 -> [_ _ w303]
              tunnel: w244 -> [_ _ w302]
              frame 17301505 {
                w279 = T13 0 items=["Grayscale (U8)", "Grayscale (I16)", "Grayscale (SGL)", "Complex (CSG)", "RGB (U32)", "HSL (U32)", "RGB (U64)", "Grayscale (U16)"] ("Image Type")
                n167 = property on="nHeight" class="DigNum (strict)"() -> ("Value"=w275:u32)  [unwired: 2 in, 2 out]
                n168 = property on="nWidth" class="DigNum (strict)"() -> ("Value"=w274:u32)  [unwired: 2 in, 2 out]
                n169 = call "IMAQ Create"("Image Name"="untitled", "Image Type"=w279) -> ("New Image"=w277:T2)  [unwired: 3 in, 1 out]
                n170 = Reshape Array(w272, w275, w274) -> (w276:u8[][])
                n171 = call "IMAQ ArrayToImage"("Image Pixels (U8)"=w276, "Image"=w277) -> ("Image Out"=w273:T2)  [unwired: 8 in, 1 out]
              }
              frame 35127316 {
                w291 = T13 4 items=["Grayscale (U8)", "Grayscale (I16)", "Grayscale (SGL)", "Complex (CSG)", "RGB (U32)", "HSL (U32)", "RGB (U64)", "Grayscale (U16)"] ("Image Type")
                n172 = Decimate 1D Array(w283) -> (w284:u8[], w285:u8[], w286:u8[])
                n173 = for {
                  tunnel: w284 -> [w292] mode=indexing
                  tunnel: w285 -> [w298] mode=indexing
                  tunnel: w286 -> [w294] mode=indexing
                  tunnel: [w293] -> w287 mode=indexing
                  tunnel: [w292] -> _ mode=indexing
                  n174 = Multiply(x=w292, y=256) -> (x*y=w299:i32)
                  n175 = Add(x=w299, y=w298) -> (x+y=w297:i32)
                  n176 = Multiply(x=w297, y=256) -> (x*y=w295:i32)
                  n177 = Add(x=w295, y=w294) -> (x+y=w293:i32)
                }
                n178 = property on="nHeight" class="DigNum (strict)"() -> ("Value"=w281:u32)  [unwired: 2 in, 2 out]
                n179 = property on="nWidth" class="DigNum (strict)"() -> ("Value"=w280:u32)  [unwired: 2 in, 2 out]
                n180 = Reshape Array(w287, w281, w280) -> (w288:i32[][])
                n181 = call "IMAQ Create"("Image Name"="untitled", "Image Type"=w291) -> ("New Image"=w289:T2)  [unwired: 3 in, 1 out]
                n182 = call "IMAQ ArrayToColorImage"("Image Pixels (U32)"=w288, "Image"=w289) -> ("Image Out"=w282:T2)  [unwired: 3 in, 1 out]
              }
              frame Default {
                w317 = T13 4 items=["Grayscale (U8)", "Grayscale (I16)", "Grayscale (SGL)", "Complex (CSG)", "RGB (U32)", "HSL (U32)", "RGB (U64)", "Grayscale (U16)"] ("Image Type")
                n183 = Compound Arithmetic op=MULTIPLY(w322, w321, u32 3 ("值")) -> (w319:u32)
                n184 = Bundle By Name(cluster="pConvertInfo In", "nWidth"=w305, "nHeight"=w304, "enSrcPixelType"=w303, "nSrcDataLen"=w302, "enDstPixelType"=u32 35127316, "nDstBufferSize"=w319) -> (w318:T5)
                n185 = property on="handle out" class="DigNum (strict)"() -> ("Value"=w325:u64)  [unwired: 2 in, 2 out]
                n186 = Initialize Array(u8 0 ("元素"), w319) -> (w324:u8[])
                n187 = call "ConvertPixelType.vi"("handle"=w325, "pSrcData"=w301, "pDstBuf In"=w324, "pConvertInfo In"=w318) -> ("pDstBuf Out"=w309:u8[])  [unwired: 7 in, 4 out]
                n188 = Decimate 1D Array(w309) -> (w310:u8[], w311:u8[], w312:u8[])
                n189 = for {
                  tunnel: w310 -> [w328] mode=indexing
                  tunnel: w311 -> [w334] mode=indexing
                  tunnel: w312 -> [w330] mode=indexing
                  tunnel: [w329] -> w313 mode=indexing
                  tunnel: [w328] -> _ mode=indexing
                  n190 = Multiply(x=w328, y=256) -> (x*y=w335:i32)
                  n191 = Add(x=w335, y=w334) -> (x+y=w333:i32)
                  n192 = Multiply(x=w333, y=256) -> (x*y=w331:i32)
                  n193 = Add(x=w331, y=w330) -> (x+y=w329:i32)
                }
                n194 = property on="nHeight" class="DigNum (strict)"() -> ("Value"=w308:u32)  [unwired: 2 in, 2 out]
                n195 = property on="nWidth" class="DigNum (strict)"() -> ("Value"=w307:u32)  [unwired: 2 in, 2 out]
                n196 = Reshape Array(w313, w308, w307) -> (w314:i32[][])
                n197 = call "IMAQ Create"("Image Name"="untitled", "Image Type"=w317) -> ("New Image"=w315:T2)  [unwired: 3 in, 1 out]
                n198 = call "IMAQ ArrayToColorImage"("Image Pixels (U32)"=w314, "Image"=w315) -> ("Image Out"=w306:T2)  [unwired: 3 in, 1 out]
              }
            }
            "Image" <- w255
            "pFrameInfoEx out" <- w254
          }
        }
      }
    }
  }
